vi "FE to Joules.vi"(5 "FE":dbl) -> (2 "J":dbl)   [LabVIEW 2021]
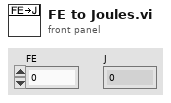
[diagram p1: front panel]
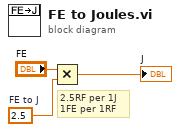
[diagram p0: block diagram]
diagram:
  w3 = 2.5  # FE to J
  # "2.5RF per 1J\n1FE per 1RF"
  n1 = Multiply(x="FE", y=w3) -> (x*y=→"J":dbl)
